vi "Create.vi"(8 "error in (no error)":errorcluster, 10 "VI":refnum<vi>) -> (0 "error out":errorcluster, 3 "Call Out":refnum<class "VI Server VI Call.lvclass">)   [LabVIEW 2020, in "VI Server VI Call.lvclass"]
uses:
  VI Server VI Call.lvclass
  VI Server VI Call.lvclass/VI Server VI Call.ctl
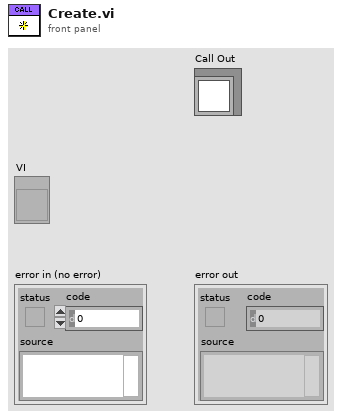
[diagram p1: front panel]
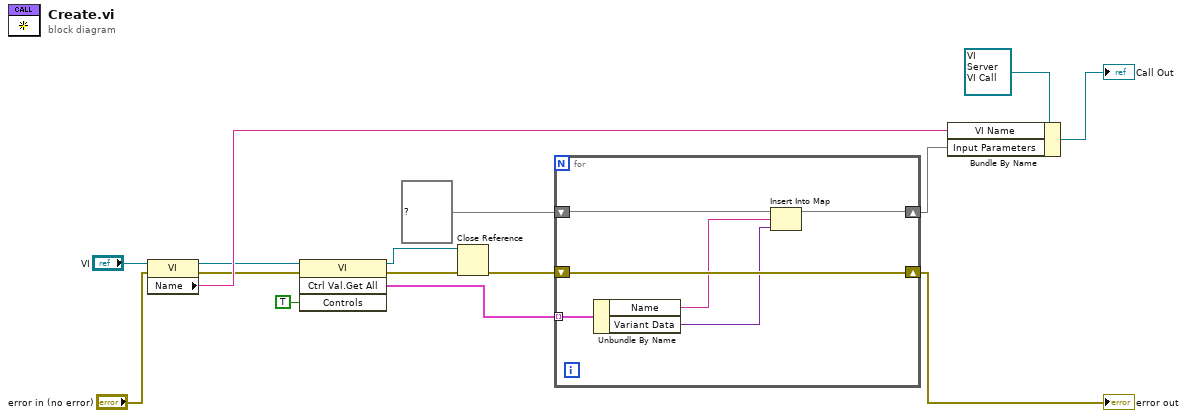
[diagram p0: block diagram]
diagram:
  n1 = property class="VI"(reference="VI", error in="error in (no error)") -> (reference out=w7:refnum<vi>, error out=w3:errorcluster, "Name"=w8:string)
  n2 = invoke class="VI" method="Ctrl Val.Get All"(reference=w7, error in=w3, "Controls"=TRUE) -> (reference out=w1:refnum<vi>, error out=w6:errorcluster, "Get All Control Values Variant"=w4:cluster{"Name":string, "Variant Data":variant}[])  [unwired: 1 in, 1 out]
  n3 = Close Reference(reference=w1, error in (no error)=w6) -> (error out=w2:errorcluster)
  n4 = for {
    shift-right: [w20] -> w9
    shift-left: map{string, variant} {} ("map") -> [w21]
    shift-right: [w19] -> w12
    shift-left: w2 -> [w19]
    tunnel: w4 -> [w18] mode=indexing
    n5 = Unbundle By Name(w18) -> ("Name"=w17:string, "Variant Data"=w16:variant)
    n6 = Insert Into Map(map in=w21, key=w17, value=w16) -> (map out=w20:map{string, variant})  [unwired: 2 out]
  }
  "error out" <- w12
  n7 = Bundle By Name(cluster=refnum<class "VI Server VI Call.lvclass"> refnum ("Call"), "VI Name"=w8, "Input Parameters"=w9) -> (→"Call Out":refnum<class "VI Server VI Call.lvclass">)
